vi "Number of Attempts.vi"() -> ()   [LabVIEW 2023]
panel:
  out "Числа, които не съвпадат":u64[](array[numeric])
  out "Съвпадащи числа":u64[](array[numeric])
  in  "Съвпадащи Числа":u64
  out "Брой опити":i32
  in  "Резултат":u64[](array[numeric])
  out "Опит":u64[](array[numeric])
  # "необходими са:"
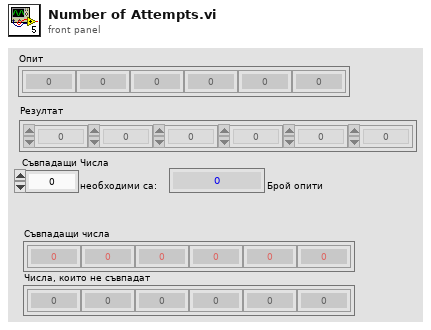
[diagram p1: front panel]
types:
  T1 = enum8{"Enabled", "Disabled", "Disabled and Grayed Out"}
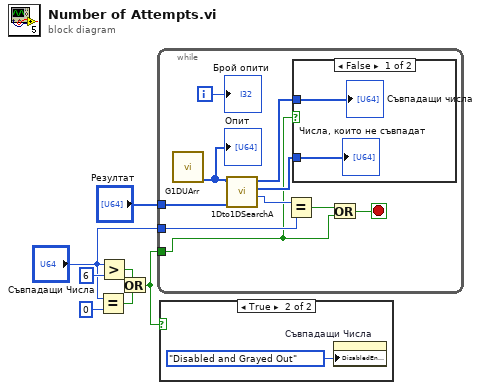
[diagram p0: block diagram]
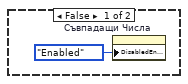
[diagram p2: hidden frame]
diagram:
  n1 = Equal?(x="Съвпадащи Числа", y=u64 0) -> (x = y?=w2:bool)
  n2 = Greater?(x="Съвпадащи Числа", y=u64 6) -> (0:w3:bool)
  n3 = Or(x=w3, y=w2) -> (x .or. y?=w1:bool)
  n4 = while {
    tunnel: "Резултат" -> [w11]
    tunnel: w1 -> [w8]
    tunnel: "Съвпадащи Числа" -> [w9]
    i -> [w17]
    stop <- w16 stop-if-true
    n5 = call "G1DUArr.vi"() -> ("1D UArr"=w10:u64[])  [unwired: 11 in]
    "Опит" <- w10
    n6 = call "1Dto1DSearchА.vi"("Array 2"=w11, "Array 1"=w10) -> ("Match El cnt"=w12:u64, "UnMatch Elements"=w14:u64[], "Match Elements"=w13:u64[])  [unwired: 6 in, 1 out]
    n7 = Equal?(x=w12, y=w9) -> (x = y?=w15:bool)
    n8 = case shown="False" w8 {
      tunnel: w14 -> [w19 _]
      tunnel: w13 -> [w18 _]
      frame False {
        "Съвпадащи числа" <- w18
        "Числа, които не съвпадат" <- w19
      }
      frame True {
      }
    }
    n9 = Or(x=w15, y=w8) -> (x .or. y?=w16:bool)
    "Брой опити" <- w17
  }
  n10 = case shown="True" w1 {
    frame False {
      n11 = property on="Съвпадащи Числа" class="DigNum (strict)"("DisabledEnum"=T1."Enabled" ("Disabled")) -> ()  [unwired: 2 in, 2 out]
    }
    frame True {
      n12 = property on="Съвпадащи Числа" class="DigNum (strict)"("DisabledEnum"=T1."Disabled and Grayed Out" ("Disabled")) -> ()  [unwired: 2 in, 2 out]
    }
  }
